vi "Vision GigE example rev B.vi"() -> ()   [LabVIEW 2014]
uses:
  <vilib>/vision/driver/IMAQdx.llb/IMAQdx Attribute Type.ctl
  <vilib>/userdefined/High Color/IMAQdx.ctl
  <vilib>/vision/driver/NI_Vision_Acquisition_Software.lvlib
  <resource>/objmgr/imaqdx.rc
panel:
  out "Attribute Name":string
  out "Attribute Information Array":T2(array[cluster])
  in  "stop":bool
  out "Running":bool
  out "error out":errorcluster
  out "Image":T3(plugin-control)
  # "This VI is example code for using the Point Grey BlackFly GigE camera\nPN BFLY-PGE-03S2C-CS.  The camera seems to require a change to\na parameter value to prevent it from posting an error....very odd!!!"
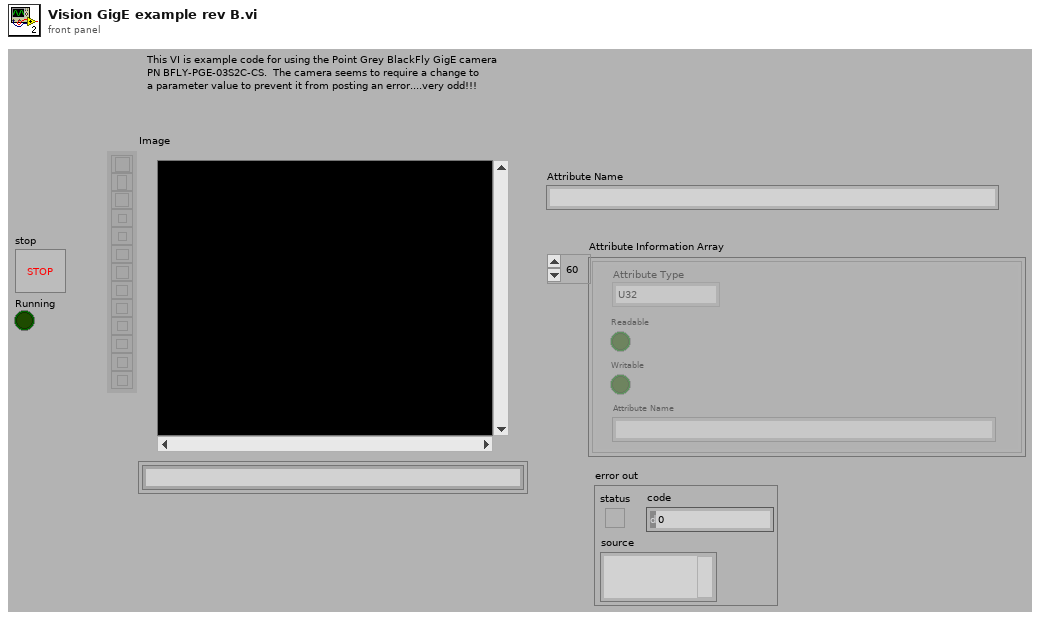
[diagram p1: front panel]
types:
  T1 = typedef "NI_Vision_Acquisition_Software.lvlib/IMAQdx Attribute Type.ctl" = enum32{"U32", "I64", "DBL", "String", "Enum", "Bool", "Command"}
  T2 = cluster{"Attribute Type":T1, "Readable":bool, "Writable":bool, "Attribute Name":string}[]
  T3 = typedef "IMAQ Image.ctl" = refnum<image>
  T4 = typedef "Image Type" = u32
  T5 = typedef "IMAQdx.ctl" = refnum<k21>
  T6 = cluster{"Attribute Type":T1, "Readable":bool, "Writable":bool, "Attribute Name":string}
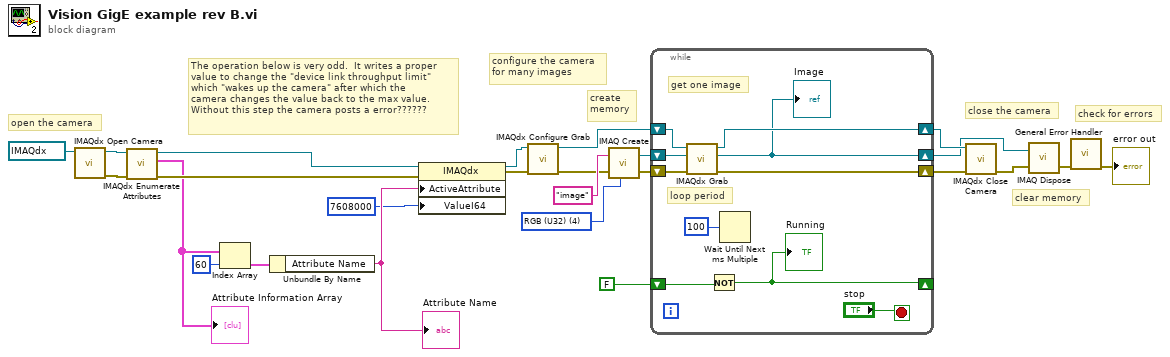
[diagram p0: block diagram]
diagram:
  w23 = T4 4 items=["Grayscale (U8)", "Grayscale (I16)", "Grayscale (SGL)", "Complex (CSG)", "RGB (U32)", "HSL (U32)", "RGB (U64)", "Grayscale (U16)"] ("Image Type")
  # "The operation below is very odd.  It writes a proper\nvalue to change the \"device link throughput limit\"\nwhich \"wakes up the camera\" after which the \ncamera changes the value back to the max value.\nWithout this step the camera posts a error??????"
  # "check for errors"
  # "clear memory"
  # "close the camera"
  # "create\nmemory"
  # "configure the camera\nfor many images"
  # "open the camera"
  n1 = call <vilib>:"IMAQdx Open Camera.vi"("Session In"=T5 "cam9") -> ("error out"=w13:errorcluster, "Session Out"=w12:T5)  [unwired: 2 in, 7 out]
  n2 = call <vilib>:"IMAQdx Enumerate Attributes.vi"("error in"=w13, "Session In"=w12) -> ("error out"=w9:errorcluster, "Attribute Information Array"=w5:T2, "Session Out"=w7:T5)  [unwired: 7 in]
  "Attribute Information Array" <- w5
  n3 = Index Array(array=w5, index=60) -> (element=w3:T6)
  n4 = Unbundle By Name(w3) -> ("Attribute Name"=w2:string)
  "Attribute Name" <- w2
  n5 = property class="IMAQdx"(reference=w7, error in=w9, "ActiveAttribute"=w2, "ValueI64"=i64 7608000) -> (reference out=w6:T5, error out=w8:errorcluster)
  n6 = call <vilib>:"IMAQdx Configure Grab.vi"("error in"=w8, "Session In"=w6) -> ("error out"=w11:errorcluster, "Session Out"=w10:T5)  [unwired: 8 out]
  n7 = call "IMAQ Create"("Image Name"="image", "Image Type"=w23, "error in (no error)"=w11) -> ("New Image"=w21:T3, "error out"=w22:errorcluster)  [unwired: 1 in, 1 out]
  n8 = while {
    shift-right: [w31] -> w20
    shift-left: w10 -> [w34]
    shift-right: [w30] -> w17
    shift-left: w21 -> [w33]
    shift-right: [w29] -> w19
    shift-left: w22 -> [w32]
    shift-right: [w27] -> _
    shift-left: FALSE -> [w28]
    stop <- "stop" stop-if-true
    # "get one image"
    # "loop period"
    n9 = call <vilib>:"IMAQdx Grab.vi"("error in"=w32, "Image In"=w33, "Session In"=w34) -> ("error out"=w29:errorcluster, "Image Out"=w30:T3, "Session Out"=w31:T5)  [unwired: 1 in, 5 out]
    "Image" <- w30
    n10 = Not(x=w28) -> (.not. x?=w27:bool)
    "Running" <- w27
    n11 = Wait Until Next ms Multiple(millisecond multiple=u32 100 ("milliseconds to wait")) -> ()  [unwired: 1 out]
  }
  n12 = call <vilib>:"IMAQdx Close Camera.vi"("error in"=w19, "Session In"=w20) -> ("error out"=w18:errorcluster)  [unwired: 9 out]
  n13 = call "IMAQ Dispose"("Image"=w17, "error in (no error)"=w18) -> ("error out"=w16:errorcluster)  [unwired: 1 in, 3 out]
  n14 = call <vilib>:"General Error Handler.vi"("error in (no error)"=w16) -> ("error out"=→"error out":errorcluster)  [unwired: 2 in, 12 out]
